vi "GV-EventsProcessing.vi"(8 "error in (no error)":errorcluster, 11 "Gviewer in":refnum<class "Gviewer.lvclass">) -> (0 "error out":errorcluster, 3 "Gviewer out":refnum<class "Gviewer.lvclass">)   [LabVIEW 2020, in "Sgraph_lib_V1.lvlib" / "Gviewer.lvclass"]
doc: "Andre Koelewijn, 1 may 2021\n\nProcess the timed events in the idle loop of the graph application."
uses:
  Gviewer.lvclass
  Gviewer.lvclass/Gviewer.ctl
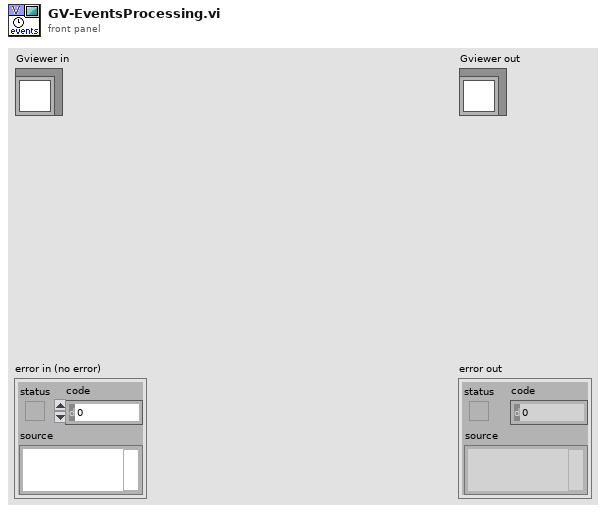
[diagram p1: front panel]
types:
  T1 = typedef "Sgraph_lib_V1.lvlib/Gviewer.lvclass/AttrIdleTimedEvents.ctl" = cluster{"UpdateToolButtons":timestamp}
  T2 = typedef "Sgraph_lib_V1.lvlib/Gviewer.lvclass/Typedef_ZoomEvent.ctl" = cluster{"Time-Start":timestamp, "Time-End":timestamp, "TimeSpan(sec)":dbl, "Live":T3, "SelProperties":T4[], "Time Stamp":timestamp}
  T3 = typedef "Sgraph_lib_V1.lvlib/Gviewer.lvclass/Typedef_Live.ctl" = enum16{"Live View", "Freeze"}
  T4 = typedef "Sgraph_lib_V1.lvlib/Gviewer.lvclass/Typedef_SelProperties.ctl" = cluster{"Color":u32, "LineType":T5, "max":dbl, "min":dbl}
  T5 = typedef "Sgraph_lib_V1.lvlib/Gviewer.lvclass/Typedef_LineType.ctl" = enum16{"num_bare", "num_MinMax_Area", "num_MinMax_Lines", "num_MinMax_Forfor", "num_Max_Area", "num_Max_Line", "num_Max_Forfor", "num_Min_Area", "num_Min_Line", "num_Min_Fosfor", "Boolean_Line_01", "Boolean_Area_01", "Boolean_Fosfor_01", "Boolean_Line_TF", "Boolean_Area_TF", "Boolean_Fosfor_TF", "Boolean_OnOff_Line", "Boolean_OnOff_Area", "Boolean_OnOff_Fosfor", "Boolean_spare", "StringEvent_Line", "StringEvent_TimeLine"}
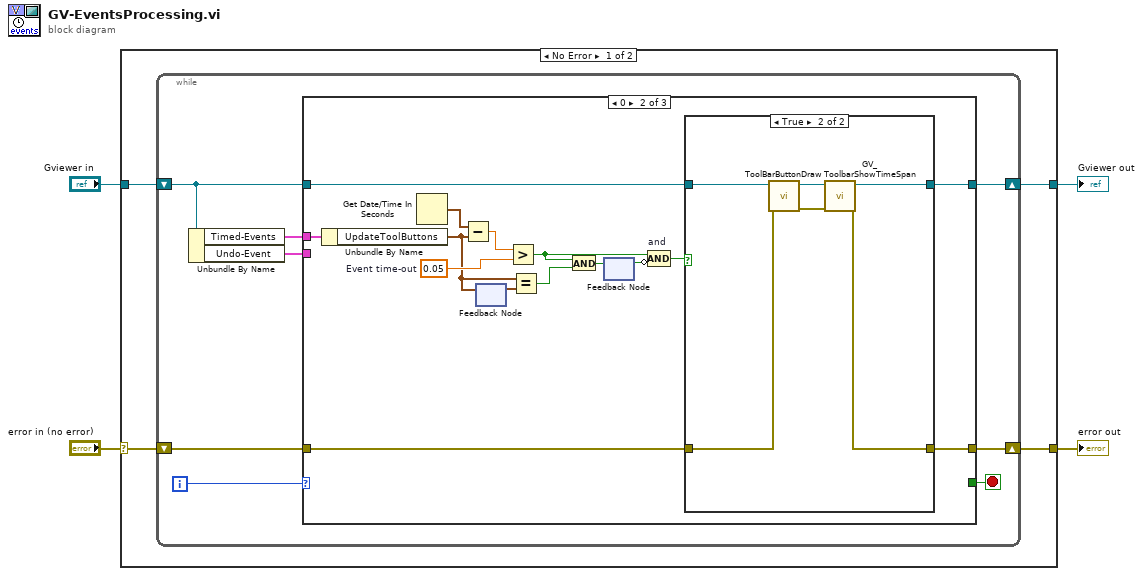
[diagram p0: block diagram]
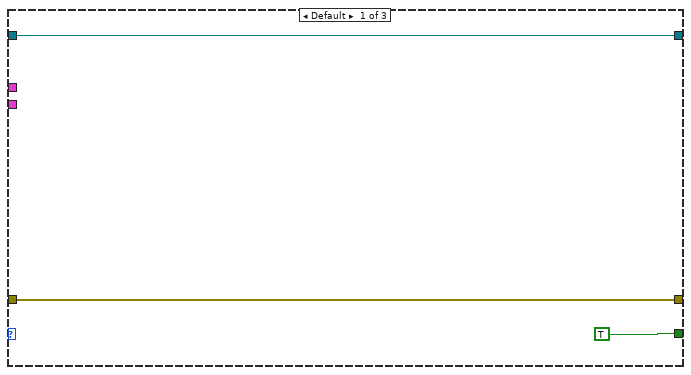
[diagram p2: hidden frame]
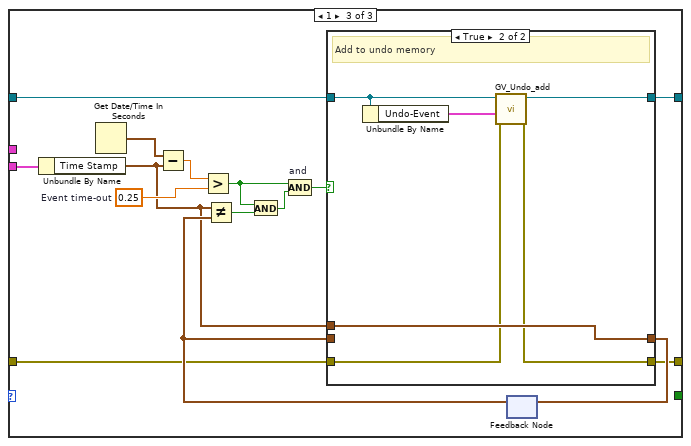
[diagram p4: hidden frame]
diagram:
  n1 = case shown="No Error" "error in (no error)" {
    selector: "error in (no error)" -> [w8 w68]
    tunnel: [w5 w68] -> w3
    tunnel: [w6 w67] -> w1
    tunnel: "Gviewer in" -> [w7 w67]
    frame No Error {
      n2 = while {
        shift-right: [w13] -> w6
        shift-left: w7 -> [w12]
        shift-right: [w9] -> w5
        shift-left: w8 -> [w14]
        i -> [w16]
        stop <- w15 stop-if-true
        n3 = Unbundle By Name(w12) -> ("Timed-Events"=w11:T1, "Undo-Event"=w10:T2)
        n4 = case shown="0" w16 {
          tunnel: [TRUE _ _] -> w15
          tunnel: w14 -> [w18 w29 w44]
          tunnel: w12 -> [w17 w27 w46]
          tunnel: [w17 w26 w45] -> w13
          tunnel: w11 -> [_ w34 _]
          tunnel: w10 -> [_ _ w57]
          tunnel: [w18 w28 w43] -> w9
          frame Default {
          }
          frame 0 {
            w31 = 0.05  # Event time-out
            n5 = Unbundle By Name(w34) -> ("UpdateToolButtons"=w24:timestamp)
            n6 = Get Date/Time In Seconds() -> (seconds since 1Jan1904=w33:timestamp)
            n7 = Subtract(x=w33, y=w24) -> (x-y=w32:dbl)
            n8 = feedback #1() -> (w25:timestamp)  [unwired: 1 in]
            n9 = feedback-in #1(w24) -> ()
            n10 = Greater?(x=w32, y=w31) -> (0:w23:bool)
            n11 = Equal?(x=w24, y=w25) -> (x = y?=w22:bool)
            n12 = And(x=w23, y=w22) -> (x .and. y?=w21:bool)
            n13 = feedback-in #2(w21) -> ()
            n14 = feedback #2() -> (w30:bool)  [unwired: 1 in]
            n15 = Compound Arithmetic op=AND "and"(w23, invert w30) -> (w20:bool)
            n16 = case shown="True" w20 {
              tunnel: [w36 w37] -> w28
              tunnel: w29 -> [w36 w41]
              tunnel: [w35 w39] -> w26
              tunnel: w27 -> [w35 w42]
              frame False {
              }
              frame True {
                n17 = call "ToolBarButtonDraw.vi"("error in (no error)"=w41, "Gviewer in"=w42) -> ("error out"=w38:errorcluster, "Gviewer out"=w40:refnum<class "Gviewer.lvclass">)  [unwired: 8 in]
                n18 = call "GV_ToolbarShowTimeSpan.vi"("error in (no error)"=w38, "Gviewer in"=w40) -> ("error out"=w37:errorcluster, "Gviewer out"=w39:refnum<class "Gviewer.lvclass">)  [unwired: 7 in, 1 out]
              }
            }
          }
          frame 1 {
            w54 = 0.25  # Event time-out
            n19 = Unbundle By Name(w57) -> ("Time Stamp"=w48:timestamp)
            n20 = Get Date/Time In Seconds() -> (seconds since 1Jan1904=w56:timestamp)
            n21 = Subtract(x=w56, y=w48) -> (x-y=w55:dbl)
            n22 = Greater?(x=w55, y=w54) -> (0:w53:bool)
            n23 = feedback #3() -> (w49:timestamp)  [unwired: 1 in]
            n24 = Not Equal?(x=w48, y=w49) -> (x != y?=w52:bool)
            n25 = And(x=w53, y=w52) -> (x .and. y?=w47:bool)
            n26 = Compound Arithmetic op=AND "and"(w53, w47) -> (w51:bool)
            n27 = case shown="True" w51 {
              tunnel: w49 -> [w60 _]
              tunnel: [w60 w66] -> w50
              tunnel: w48 -> [_ w66]
              tunnel: w46 -> [w59 w64]
              tunnel: [w59 w65] -> w45
              tunnel: w44 -> [w58 w63]
              tunnel: [w58 w62] -> w43
              frame False {
                # "no action"
              }
              frame True {
                # "Add to undo memory"
                n28 = Unbundle By Name(w64) -> ("Undo-Event"=w61:T2)
                n29 = call "GV_Undo_add.vi"("error in (no error)"=w63, "ZoomEvent"=w61, "Gviewer in"=w64) -> ("error out"=w62:errorcluster, "Gviewer out"=w65:refnum<class "Gviewer.lvclass">)  [unwired: 7 in]
              }
            }
            n30 = feedback-in #3(w50) -> ()
          }
        }
      }
    }
    frame Error {
    }
  }
  "error out" <- w3
  "Gviewer out" <- w1
